vi "Set_2G_Attach_Detach_Allowed.vi"(8 "error in (no error)":errorcluster, 10 "value":i32 min=0 max=1, 11 "Base Station":T1) -> (0 "error out":errorcluster, 3 "Output String":string)   [LabVIEW 2021]
uses:
  Controls/Base_Station_Emulator.ctl
  Controls/TCP_FGV.ctl
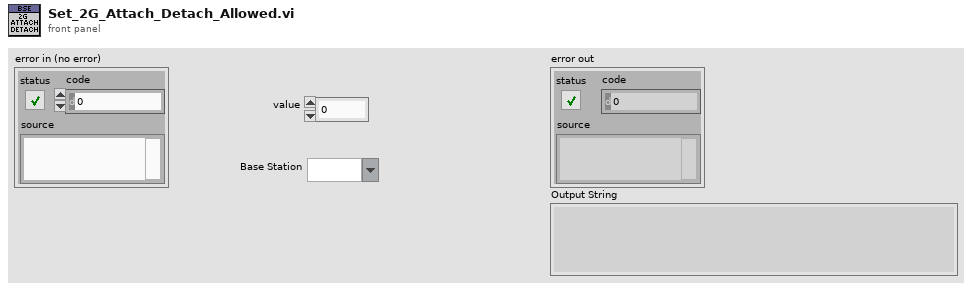
[diagram p1: front panel]
types:
  T1 = typedef "Base_Station_Emulator.ctl" = string
  T2 = typedef "TCP_FGV.ctl" = enum16{"Open", "Read", "Write", "Close"}
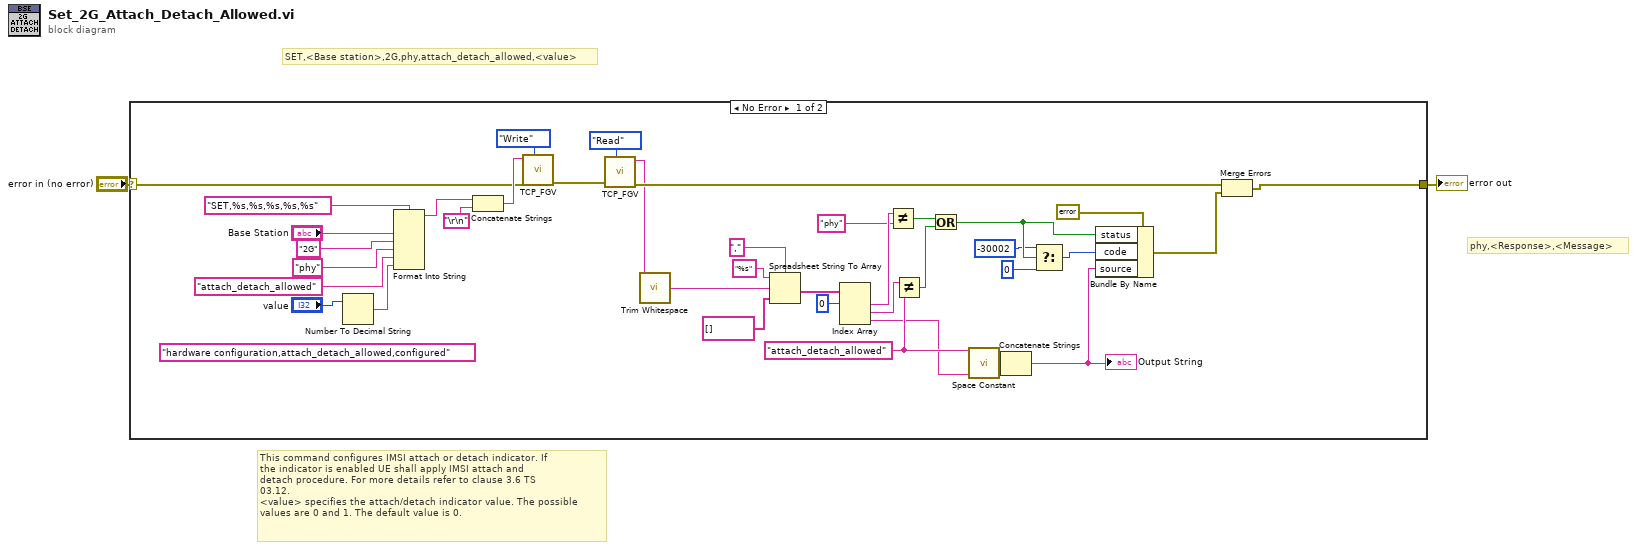
[diagram p0: block diagram]
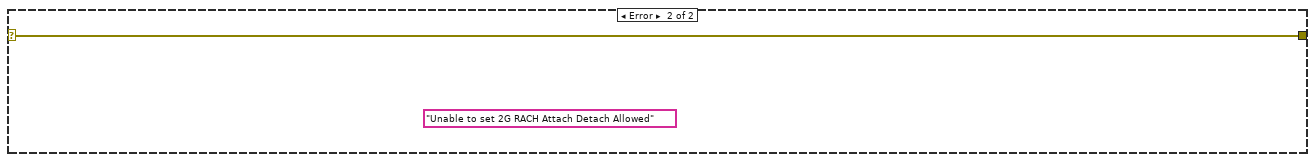
[diagram p2: hidden frame]
diagram:
  # "This command configures IMSI attach or detach indicator. If \nthe indicator is enabled UE shall apply IMSI attach and \ndetach procedure. For more details refer to clause 3.6 TS \n03.12. \n<value> specifies the attach/detach indicator value. The possible \nvalues are 0 and 1. The default value is 0."
  # "phy,<Response>,<Message>"
  # "SET,<Base station>,2G,phy,attach_detach_allowed,<value>"
  n1 = case shown="No Error" "error in (no error)" {
    selector: "error in (no error)" -> [w3 w41]
    tunnel: [w15 w41] -> w1
    frame No Error {
      (unwired) "hardware configuration,attach_detach_allowed,configured" ("format string")
      w13 = "attach_detach_allowed"
      n2 = Number To Decimal String(number="value") -> (decimal integer string=w8:string)  [unwired: 1 in]
      n3 = Format Into String(format string="SET,%s,%s,%s,%s,%s", "Base Station", "2G", "phy", "attach_detach_allowed", w8) -> (resulting string=w6:string)  [unwired: 2 in, 1 out]
      n4 = Concatenate Strings(w6, "\r\n") -> (w5:string)
      n5 = call "TCP_FGV.vi"("Command"=w5, "error in (no error)"=w3, "Operation"=TCP_FGV."Write") -> ("error out"=w16:errorcluster)  [unwired: 6 in, 1 out]
      n6 = call "TCP_FGV.vi"("error in (no error)"=w16, "Operation"=TCP_FGV."Read") -> ("Data Out"=w17:string, "error out"=w19:errorcluster)  [unwired: 7 in]
      n7 = call <vilib>:"Trim Whitespace.vi"("string"=w17) -> ("trimmed string"=w33:string)  [unwired: 1 in]
      n8 = Spreadsheet String To Array(delimiter (Tab)=",", format string="%s", spreadsheet string=w33, array type (2D Dbl)=string[] []) -> (array=w29:string[])
      n9 = Index Array(array=w29, index #1=0 ("index")) -> (element #1=w30:string, element #2=w20:string, element #3=w12:string)  [unwired: 2 in]
      n10 = Not Equal?(x=w30, y="phy" ("format string")) -> (x != y?=w31:bool)
      n11 = Not Equal?(x=w20, y=w13) -> (x != y?=w32:bool)
      n12 = Or(x=w31, y=w32) -> (x .or. y?=w34:bool)
      n13 = call <vilib>:"Space Constant.vi"() -> ("String"=w14:string)
      n14 = Concatenate Strings(w13, w14, w12) -> (w11:string)
      "Output String" <- w11
      n15 = Select(t=-30002 ("code"), s=w34, f=0 ("code")) -> (s? t:f=w35:i32)
      n16 = Bundle By Name(cluster=errorcluster {"status"=FALSE, "code"=0, "source"=""} ("error constant"), "status"=w34, "code"=w35, "source"=w11) -> (w18:errorcluster)
      n17 = Merge Errors(w19, w18) -> (w15:errorcluster)
    }
    frame Error {
      (unwired) "Unable to set 2G RACH Attach Detach Allowed" ("source")
    }
  }
  "error out" <- w1
